vi "Cholesky Factorization.vi"   [LabVIEW 2010, in "NI_AALPro.lvlib"]
doc: "Performs Cholesky factorization on a symmetric or Hermitian positive definite matrix. Wire data to the <B>A</B> input to determine the polymorphic instance to use or manually select the instance."
uses:
  NI_AALPro.lvlib
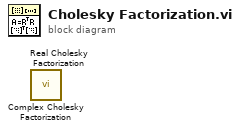
[diagram p0: block diagram]
diagram:
  n1 = call "Complex Cholesky Factorization.vi"() -> ()  [unwired: 1 in, 2 out]
  n2 = call "Real Cholesky Factorization.vi"() -> ()  [unwired: 1 in, 2 out]
